vi "CreateIndices (DNet CommandRegister Buffer).vi"(8 "error in":errorcluster[](array[cluster]), 11 "connection in":refnum<k13>[](array[refnum])) -> (0 "error out":errorcluster[](array[cluster]), 1 "Indices":i32[](array[numeric]), 2 "DNet CommandRegister Buffer":bool[](array[boolean]), 3 "connection out":refnum<k13>[](array[refnum]))   [LabVIEW 2011]
uses:
  GlobalVariables.vi
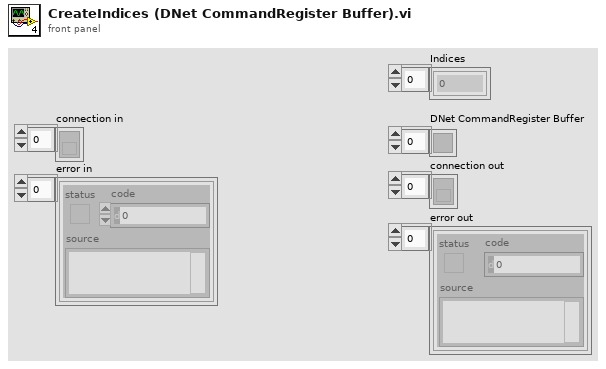
[diagram p1: front panel]
types:
  T1 = typedef "DNet CommandRegister Cluster.ctl" = cluster{"Run":bool, "Fault":bool, "DisableNetowrk":bool, "HaltScanner":bool, "Reset":bool}
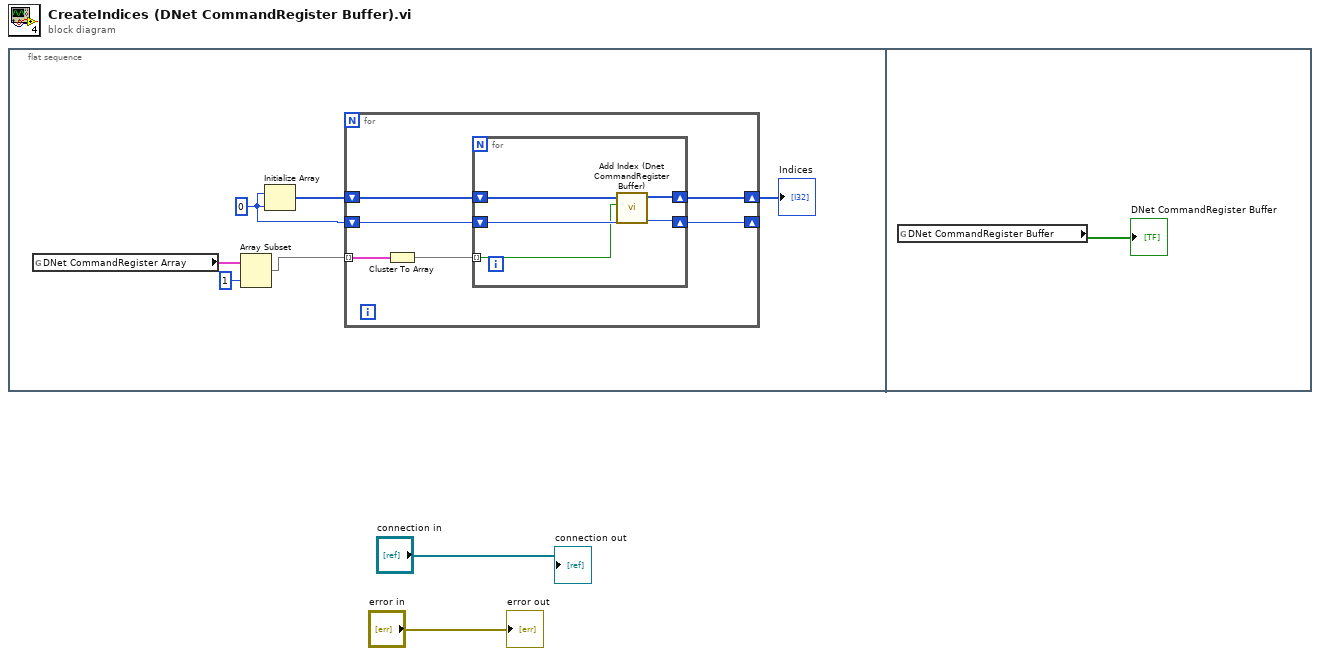
[diagram p0: block diagram]
diagram:
  n1 = flat-sequence {
    frame #0 {
      w7 = 0 ("dimension size")
      n2 = global read "GlobalVariables.vi" "DNet CommandRegister Array"() -> (w5:T1[])
      n3 = Array Subset(array=w5, index=1) -> (w3:T1[])  [unwired: 1 in]
      n4 = Initialize Array(w7, w7) -> (w8:i32[])
      n5 = for {
        tunnel: w3 -> [w14] mode=indexing
        shift-right: [w9] -> w6
        shift-left: w8 -> [w11]
        shift-right: [w10] -> _
        shift-left: w7 -> [w12]
        n6 = Cluster To Array(cluster=w14) -> (array=w13:bool[])
        n7 = for {
          tunnel: w13 -> [w15] mode=indexing
          shift-right: [w16] -> w9
          shift-left: w11 -> [w19]
          shift-right: [w17] -> w10
          shift-left: w12 -> [w18]
          n8 = call "Add Index (Dnet CommandRegister Buffer).vi"("Count"=w18, "Value"=w15, "Indices Input"=w19) -> ("Count+1"=w17:i32, "Indices Output"=w16:i32[])  [unwired: 7 in]
        }
      }
      "Indices" <- w6
    }
    frame #1 {
      n9 = global read "GlobalVariables.vi" "DNet CommandRegister Buffer"() -> (→"DNet CommandRegister Buffer":bool[])
    }
  }
  "connection out" <- "connection in"
  "error out" <- "error in"
